vi "Stop VeriStand.vi"(9 "GatewayIP":string, 10 "ProjectFilePath":path, 11 "Sequence Context":T1) -> (0 "error out":errorcluster)   [LabVIEW 2013, in "MiscHelperVIs.lvlib"]
uses:
  MiscHelperVIs.lvlib
  <vilib>/addons/TestStand/_TSLegacy.llb/LabVIEW Test - Sequence Context.ctl
  <vilib>/NI Veristand/Execution/Project/NI_VS Project ExecutionAPI.lvlib
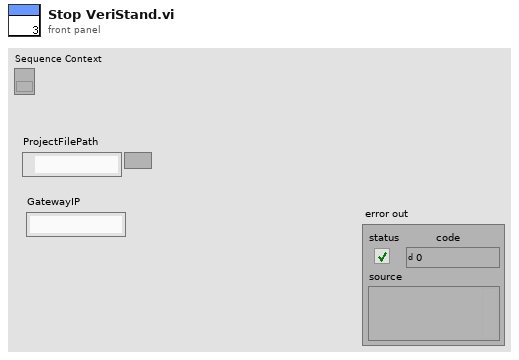
[diagram p1: front panel]
types:
  T1 = typedef "LabVIEW Test - Sequence Context.ctl" = refnum<k7>
  T2 = typedef "NI_VS Project ExecutionAPI.lvlib/Project Ref.ctl" = refnum<k24>
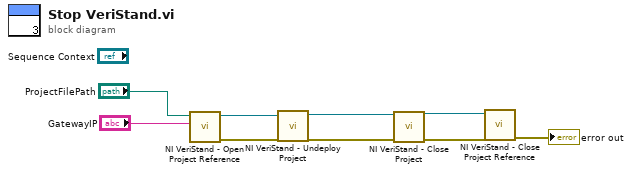
[diagram p0: block diagram]
diagram:
  n1 = call <vilib>:"NI VeriStand - Open Project Reference.vi"("Gateway IP Address (\"\": localhost)"="GatewayIP", "Project File Path"="ProjectFilePath") -> ("error out"=w6:errorcluster, "Project Ref"=w7:T2)  [unwired: 8 in]
  n2 = call <vilib>:"NI VeriStand - Undeploy Project.vi"("error in (no error)"=w6, "Project Ref in"=w7) -> ("error out"=w4:errorcluster, "Project Ref out"=w5:T2)  [unwired: 8 in]
  n3 = call <vilib>:"NI VeriStand - Close Project.vi"("error in (no error)"=w4, "Project Ref in"=w5) -> ("error out"=w3:errorcluster, "Project Ref out"=w2:T2)  [unwired: 8 in]
  n4 = call <vilib>:"NI VeriStand - Close Project Reference.vi"("error in (no error)"=w3, "Project Ref"=w2) -> ("error out"=→"error out":errorcluster)  [unwired: 9 in]
